vi "Internal Read.vi"(8 "error in (no error)":errorcluster, 10 "timeout ms":i32, 11 "WebSocket in":refnum<class "WebSocket.lvclass">) -> (0 "error out":errorcluster, 1 "Opcode":T1 items=["Cont. Frame", "Text", "Binary", "Close Frame", "Ping", "Pong"], 2 "Data":u8[](array[numeric]), 3 "WebSocket out":refnum<class "WebSocket.lvclass">)   [LabVIEW 2021, in "WebSockets.lvlib" / "WebSocket.lvclass"]
doc: "Performs a read operation and handles internal WebSockets considerations.\n\n- Will read multi-framed messages as a single read\n- Automatically responds to Ping requests\n- Generates an error on receipt of a close frame\n\nVI will return when a 'complete' frame is read or a timeout occurs.\nWebSockets 2.0.1.40\nSam Sharp - MediaMongrels Ltd\nCopyright (c) 2019, MediaMongrels Ltd"
uses:
  WebSocket.lvclass
  Opcodes.ctl
  WebSocket.lvclass/WebSocket.ctl
  Socket Read.vi
  Low-Level Write.vi
  DataLengthBytes.vi
  EncodeMaskedBytes.vi
  Socket Write.vi
  DecodeMaskedBytes.vi
  Sockets/Socket/Socket.lvclass
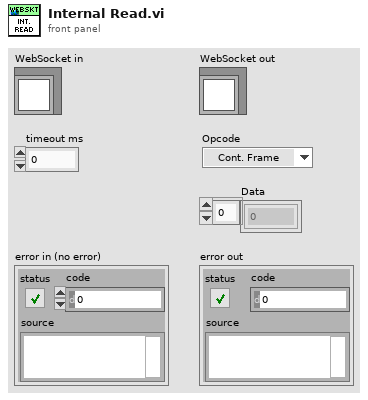
[diagram p1: front panel]
types:
  T1 = typedef "WebSockets.lvlib/WebSocket.lvclass/Opcodes.ctl" = u8
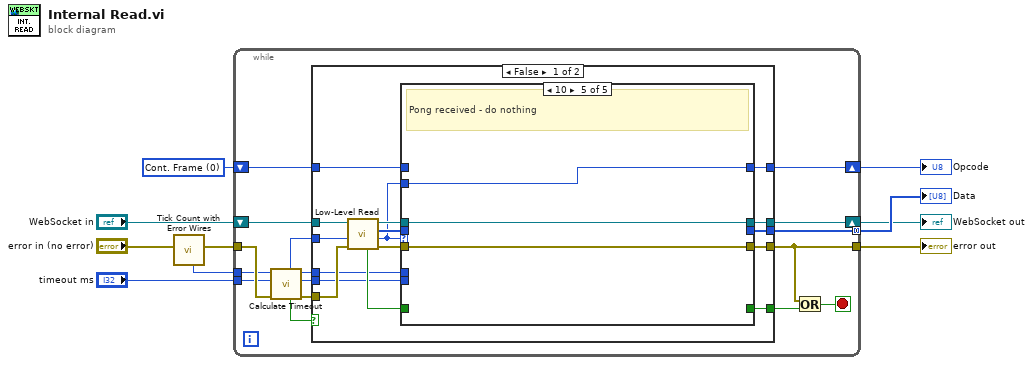
[diagram p0: block diagram]
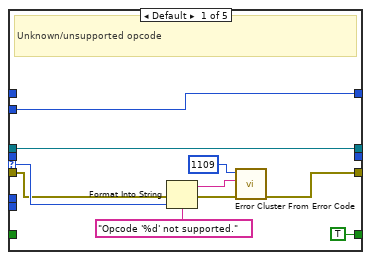
[diagram p2: hidden frame]
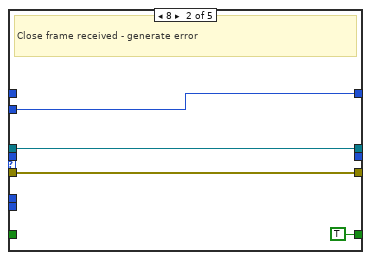
[diagram p3: hidden frame]
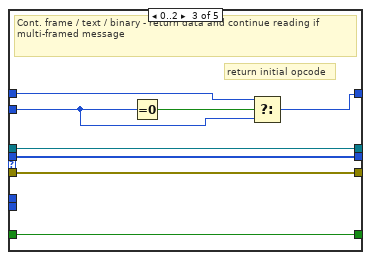
[diagram p4: hidden frame]
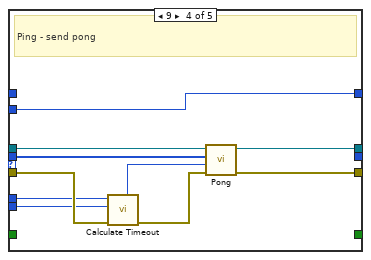
[diagram p5: hidden frame]
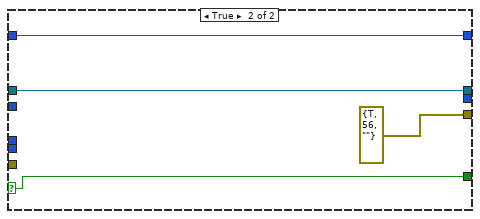
[diagram p6: hidden frame]
diagram:
  w1 = T1 0 items=["Cont. Frame", "Text", "Binary", "Close Frame", "Ping", "Pong"] ("Opcode")
  n1 = call "Tick Count with Error Wires.vi"("error in (no error)"="error in (no error)") -> ("error out"=w3:errorcluster, "millisecond timer value"=w2:u32)  [unwired: 9 in]
  n2 = while {
    tunnel: w3 -> [w16]
    tunnel: "timeout ms" -> [w12]
    tunnel: [w22] -> w8
    shift-right: [w21] -> w7
    shift-left: "WebSocket in" -> [w24]
    tunnel: [w20] -> w10 mode=concatenating
    shift-right: [w18] -> w9
    shift-left: w1 -> [w17]
    tunnel: w2 -> [w13]
    stop <- w23 stop-if-true
    n3 = call "Calculate Timeout.vi"("error in (no error)"=w16, "timeout ms"=w12, "t0"=w13) -> ("error out"=w15:errorcluster, "Elapsed?"=w11:bool, "new timeout ms"=w14:i32)  [unwired: 6 in]
    n4 = case shown="False" w11 {
      selector: w11 -> [_ w77]
      tunnel: w24 -> [w40 w78]
      tunnel: [w38 errorcluster {"status"=TRUE, "code"=56, "source"=""} ("error out")] -> w22
      tunnel: [w35 w78] -> w21
      tunnel: [w34 _] -> w20
      tunnel: [w33 w77] -> w19
      tunnel: [w31 w79] -> w18
      tunnel: w17 -> [w29 w79]
      tunnel: w15 -> [w28 _]
      tunnel: w14 -> [w27 _]
      tunnel: w13 -> [w26 _]
      tunnel: w12 -> [w25 _]
      frame False {
        n5 = call "Low-Level Read.vi"("error in (no error)"=w28, "timeout ms (5000)"=w27, "WebSockets in"=w40) -> ("error out"=w39:errorcluster, "Opcode"=w30:T1, "Data"=w36:u8[], "WebSockets out"=w37:refnum<class "WebSocket.lvclass">, "Finished?"=w32:bool)  [unwired: 4 in]
        n6 = case shown="10" w30 {
          selector: w30 -> [w45 _ _ _ _]
          tunnel: w39 -> [w44 w53 w61 w67 w74]
          tunnel: [w43 w53 w61 w70 w74] -> w38
          tunnel: w37 -> [w42 w52 w62 w72 w75]
          tunnel: w36 -> [_ _ w60 w71 _]
          tunnel: [w42 w52 w62 w69 w75] -> w35
          tunnel: [_ _ w60 _ _] -> w34
          tunnel: [TRUE ("Finished?") TRUE ("Finished?") w59 _ _] -> w33
          tunnel: w32 -> [_ _ w59 _ _]
          tunnel: [w41 w51 w57 w68 w73] -> w31
          tunnel: w30 -> [w41 w51 w55 w68 w73]
          tunnel: w29 -> [_ _ w56 _ _]
          tunnel: w26 -> [_ _ _ w66 _]
          tunnel: w25 -> [_ _ _ w65 _]
          frame Default {
            # "Unknown/unsupported opcode"
            n7 = Format Into String(format string="Opcode '%d' not supported.", error in=w44, w45) -> (resulting string=w48:string, error out=w49:errorcluster)  [unwired: 1 in]
            n8 = call <vilib>:"Error Cluster From Error Code.vi"("error in (no error)"=w49, "error message (\"\")"=w48, "error code (0)"=1109) -> ("error out"=w43:errorcluster)  [unwired: 6 in]
          }
          frame 8 {
            # "Close frame received - generate error"
          }
          frame 0..2 {
            # "return initial opcode"
            # "Cont. frame / text / binary - return data and continue reading if multi-framed message"
            n9 = Equal To 0?(x=w55) -> (x = 0?=w58:bool)
            n10 = Select(t=w56, s=w58, f=w55) -> (s? t:f=w57:T1)
          }
          frame 9 {
            # "Ping - send pong"
            n11 = call "Calculate Timeout.vi"("error in (no error)"=w67, "timeout ms"=w65, "t0"=w66) -> ("error out"=w64:errorcluster, "new timeout ms"=w63:i32)  [unwired: 6 in, 1 out]
            n12 = call "Pong.vi"("error in (no error)"=w64, "timeout ms (5000)"=w63, "Ping Payload"=w71, "WebSocket in"=w72) -> ("error out"=w70:errorcluster, "WebSocket out"=w69:refnum<class "WebSocket.lvclass">)  [unwired: 5 in, 1 out]
          }
          frame 10 {
            # "Pong received - do nothing"
          }
        }
      }
      frame True {
      }
    }
    n13 = Or(x=w22, y=w19) -> (x .or. y?=w23:bool)
  }
  "Data" <- w10
  "Opcode" <- w9
  "error out" <- w8
  "WebSocket out" <- w7
